vi "TypecastControls.vi"(0 "Controls[]":refnum<vi>[](array[refnum]), 5 "Control Name":string, 9 "Control Path In":string[](array[string]), 11 "error In":errorcluster) -> (4 "Sub Controls[]":refnum<vi>[](array[refnum]), 10 "Control Path Out":string[](array[string]), 15 "error out":errorcluster)   [LabVIEW 2016, in "Drona.lvlib" / "GetControlRef.lvlib"]
doc: "Typecasts the control to its respective class and gives the reference of the controls inside it."
uses:
  GetControlRef.lvlib
  Drona.lvlib
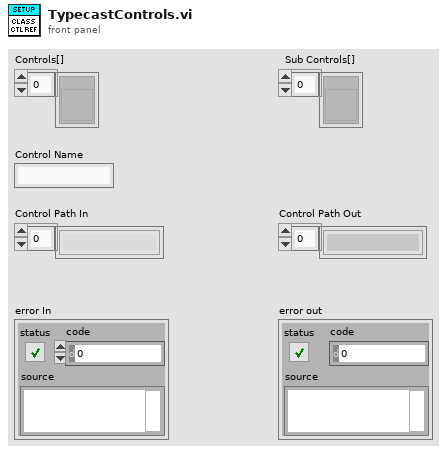
[diagram p1: front panel]
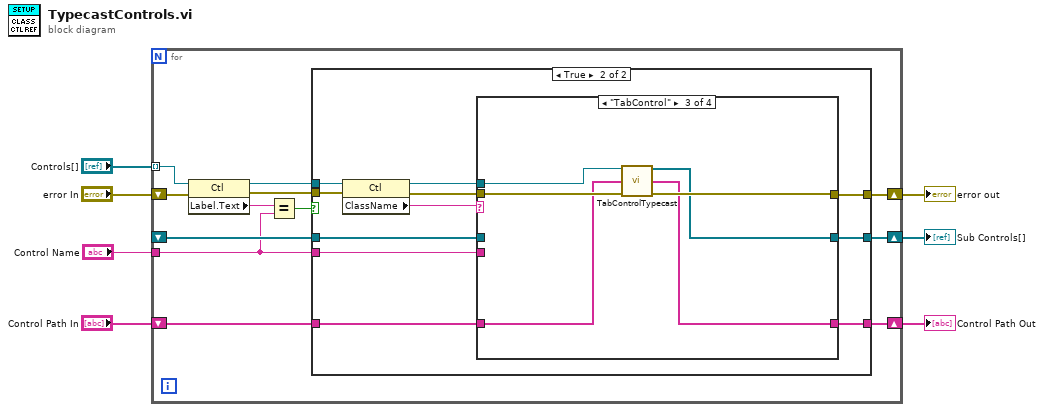
[diagram p0: block diagram]
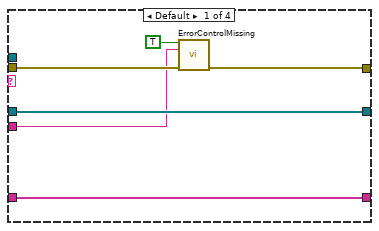
[diagram p3: hidden frame]
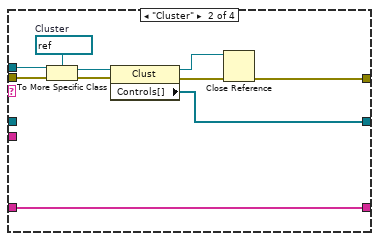
[diagram p4: hidden frame]
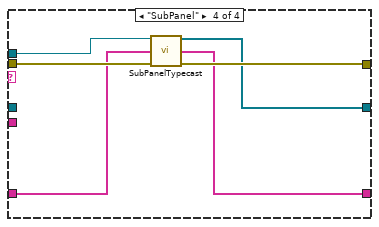
[diagram p5: hidden frame]
diagram:
  n1 = for {
    tunnel: "Controls[]" -> [w19] mode=indexing
    tunnel: "Control Name" -> [w8]
    shift-right: [w14] -> w3
    shift-left: _ -> [w13]
    shift-right: [w12] -> w4
    shift-left: "error In" -> [w11]
    shift-right: [w9] -> w1
    shift-left: "Control Path In" -> [w10]
    n2 = property class="Ctl"(reference=w19, error in=w11) -> (reference out=w15:refnum<vi>, error out=w16:errorcluster, "Label.Text"=w18:string)
    n3 = Equal?(x=w18, y=w8) -> (x = y?=w17:bool)
    n4 = case shown="True" w17 {
      tunnel: w16 -> [w21 w33]
      tunnel: w15 -> [_ w32]
      tunnel: [w22 w28] -> w14
      tunnel: w13 -> [w22 w26]
      tunnel: [w21 w27] -> w12
      tunnel: w10 -> [w20 w25]
      tunnel: [w20 w24] -> w9
      tunnel: w8 -> [_ w23]
      frame False {
      }
      frame True {
        n5 = property class="Ctl"(reference=w32, error in=w33) -> (reference out=w29:refnum<vi>, error out=w30:errorcluster, "ClassName"=w31:string)
        n6 = case shown="\"TabControl\"" w31 {
          tunnel: w30 -> [w37 w49 w55 w61]
          tunnel: w29 -> [_ w48 w54 w57]
          tunnel: [w39 w44 w50 w56] -> w28
          tunnel: [w36 w42 w52 w60] -> w27
          tunnel: w26 -> [w39 _ _ _]
          tunnel: w25 -> [w38 w40 w53 w59]
          tunnel: [w38 w40 w51 w58] -> w24
          tunnel: w23 -> [w34 _ _ _]
          frame Default {
            n7 = call "ErrorControlMissing.vi"("Create Error?"=TRUE, "Control Name"=w34, "error in"=w37) -> ("error out"=w36:errorcluster)  [unwired: 12 in]
          }
          frame "Cluster" {
            w47 = refnum<vi> refnum  # Cluster
            n8 = To More Specific Class(target class=w47, reference=w48, error in=w49) -> (specific class reference=w46:refnum<vi>, error out=w45:errorcluster)
            n9 = property class="Clust"(reference=w46, error in=w45) -> (reference out=w41:refnum<vi>, error out=w43:errorcluster, "Controls[]"=w44:refnum<vi>[])
            n10 = Close Reference(reference=w41, error in (no error)=w43) -> (error out=w42:errorcluster)
          }
          frame "TabControl" {
            n11 = call "TabControlTypecast.vi"("Ctl Refnum"=w54, "Control Path In"=w53, "Error In"=w55) -> ("Controls[]"=w50:refnum<vi>[], "Control Path Out"=w51:string[], "Error Out"=w52:errorcluster)  [unwired: 10 in]
          }
          frame "SubPanel" {
            n12 = call "SubPanelTypecast.vi"("Ctl Refnum"=w57, "Control Path In"=w59, "Error In"=w61) -> ("Controls[]"=w56:refnum<vi>[], "Control Path Out"=w58:string[], "Error Out"=w60:errorcluster)  [unwired: 10 in]
          }
        }
      }
    }
  }
  "error out" <- w4
  "Sub Controls[]" <- w3
  "Control Path Out" <- w1
